vi "Create Information Window String.vi"(9 "Current Network Index":i32, 10 "Net Data":T3, 11 "Information Window Reference":refnum<vi>) -> ()   [LabVIEW 2019]
uses:
  Advanced Search.llb/Terminal Filter Output.ctl
  Advanced Search.llb/Terminals within Selection and GObject.ctl
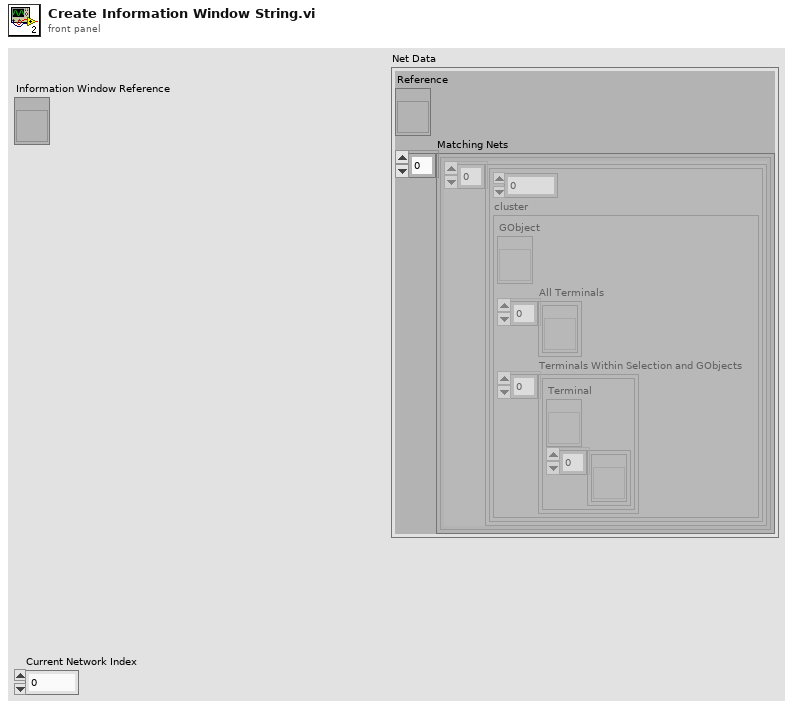
[diagram p1: front panel]
types:
  T1 = typedef "Terminal Filter Output.ctl" = cluster{"GObject":refnum<vi>, "All Terminals":refnum<vi>[], "Terminals Within Selection and GObjects":T2[]}
  T2 = typedef "Terminals within Selection and GObject.ctl" = cluster{"Terminal":refnum<vi>, "Attached GObjects":refnum<vi>[]}
  T3 = cluster{"Reference":refnum<vi>, "Matching Nets":cluster{cluster{i32, "cluster":T1}[]}[]}
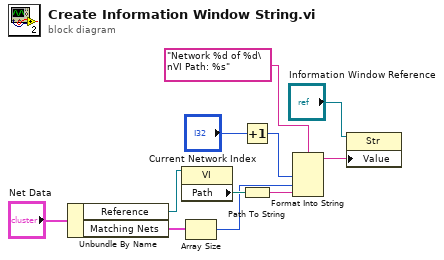
[diagram p0: block diagram]
diagram:
  n1 = Unbundle By Name("Net Data") -> ("Reference"=w1:refnum<vi>, "Matching Nets"=w2:cluster{cluster{i32, "cluster":T1}[]}[])
  n2 = property class="VI"(reference=w1) -> ("Path"=w10:path)  [unwired: 1 in, 2 out]
  n3 = Array Size(array=w2) -> (size(s)=w8:i32)
  n4 = Increment(x="Current Network Index") -> (x+1=w9:i32)
  n5 = Path To String(path=w10) -> (string=w11:string)
  n6 = Format Into String(format string="Network %d of %d\nVI Path: %s", w9, w8, w11) -> (resulting string=w6:string)  [unwired: 2 in, 1 out]
  n7 = property class="Str"(reference="Information Window Reference", "Value"=w6) -> ()  [unwired: 1 in, 2 out]
